vi "Mice staircase kinematics - MAIN.vi"() -> ()   [LabVIEW 2020]
panel:
  in  "FPS":dbl
  in  "Synergy data":string
  in  "Path length data":string
  in  "Velocity, acceleration graphs":string
  in  "Velocity, acceleration, smoothness data":string
  in  "Angle graphs":string
  in  "Angle data":string
  in  "Position graph":string
  in  "Position data":string
  out "Shoulder-Elbow angle data":dbl[][](array[numeric])
  out "Vel, Acc data":dbl[][](array[numeric])
  out "Angle-angle synergygrap":i32[][](array[numeric])
  out "Angle-angle synergy":dbl[][](array[numeric])
  out "Pos, Neg increments Position":dbl[][](array[numeric])
  out "Synergy Graph":i32[][](array[numeric])
  out "Synergy%":i32[][](array[numeric])
  out "Vel, Accel RMS":dbl[][](array[numeric])
  out "Path length data":dbl[][](array[numeric])
  in  "Step":dbl
  in  "Animal Number":dbl
  out "#Crossings":i32[][](array[numeric])
  out "Velocity-Acceleration graphs":dbl[][](array[numeric])
  out "Raw position":dbl[][](array[numeric])
  out "Pos, Neg increments":dbl[][](array[numeric])
  out "Elbow CircStat":dbl[](array[numeric])
  out "Shoulder CircStat Counterclockwise":dbl[](array[numeric])
  out "Angle RMS":dbl[][](array[numeric])
  out "Angle mean subtracted (output)":dbl[][](array[numeric])
  out "RMS":dbl[][](array[numeric])
  out "Normalized Position":dbl[][](array[numeric])
  out "Position (output)":dbl[][](array[numeric])
  # "The post-stroke hemiplegic rodent evaluation"
  # "FILE NAMES (DATA)"
  # "MAIN CONTROLS"
  # "DATA"
  # "FILE NAMES (GRAPHS)"
  # "GRAPHS"
  # "LabVIEW code by Gustavo Balbinot & Clarissa Pedrini Schuch"
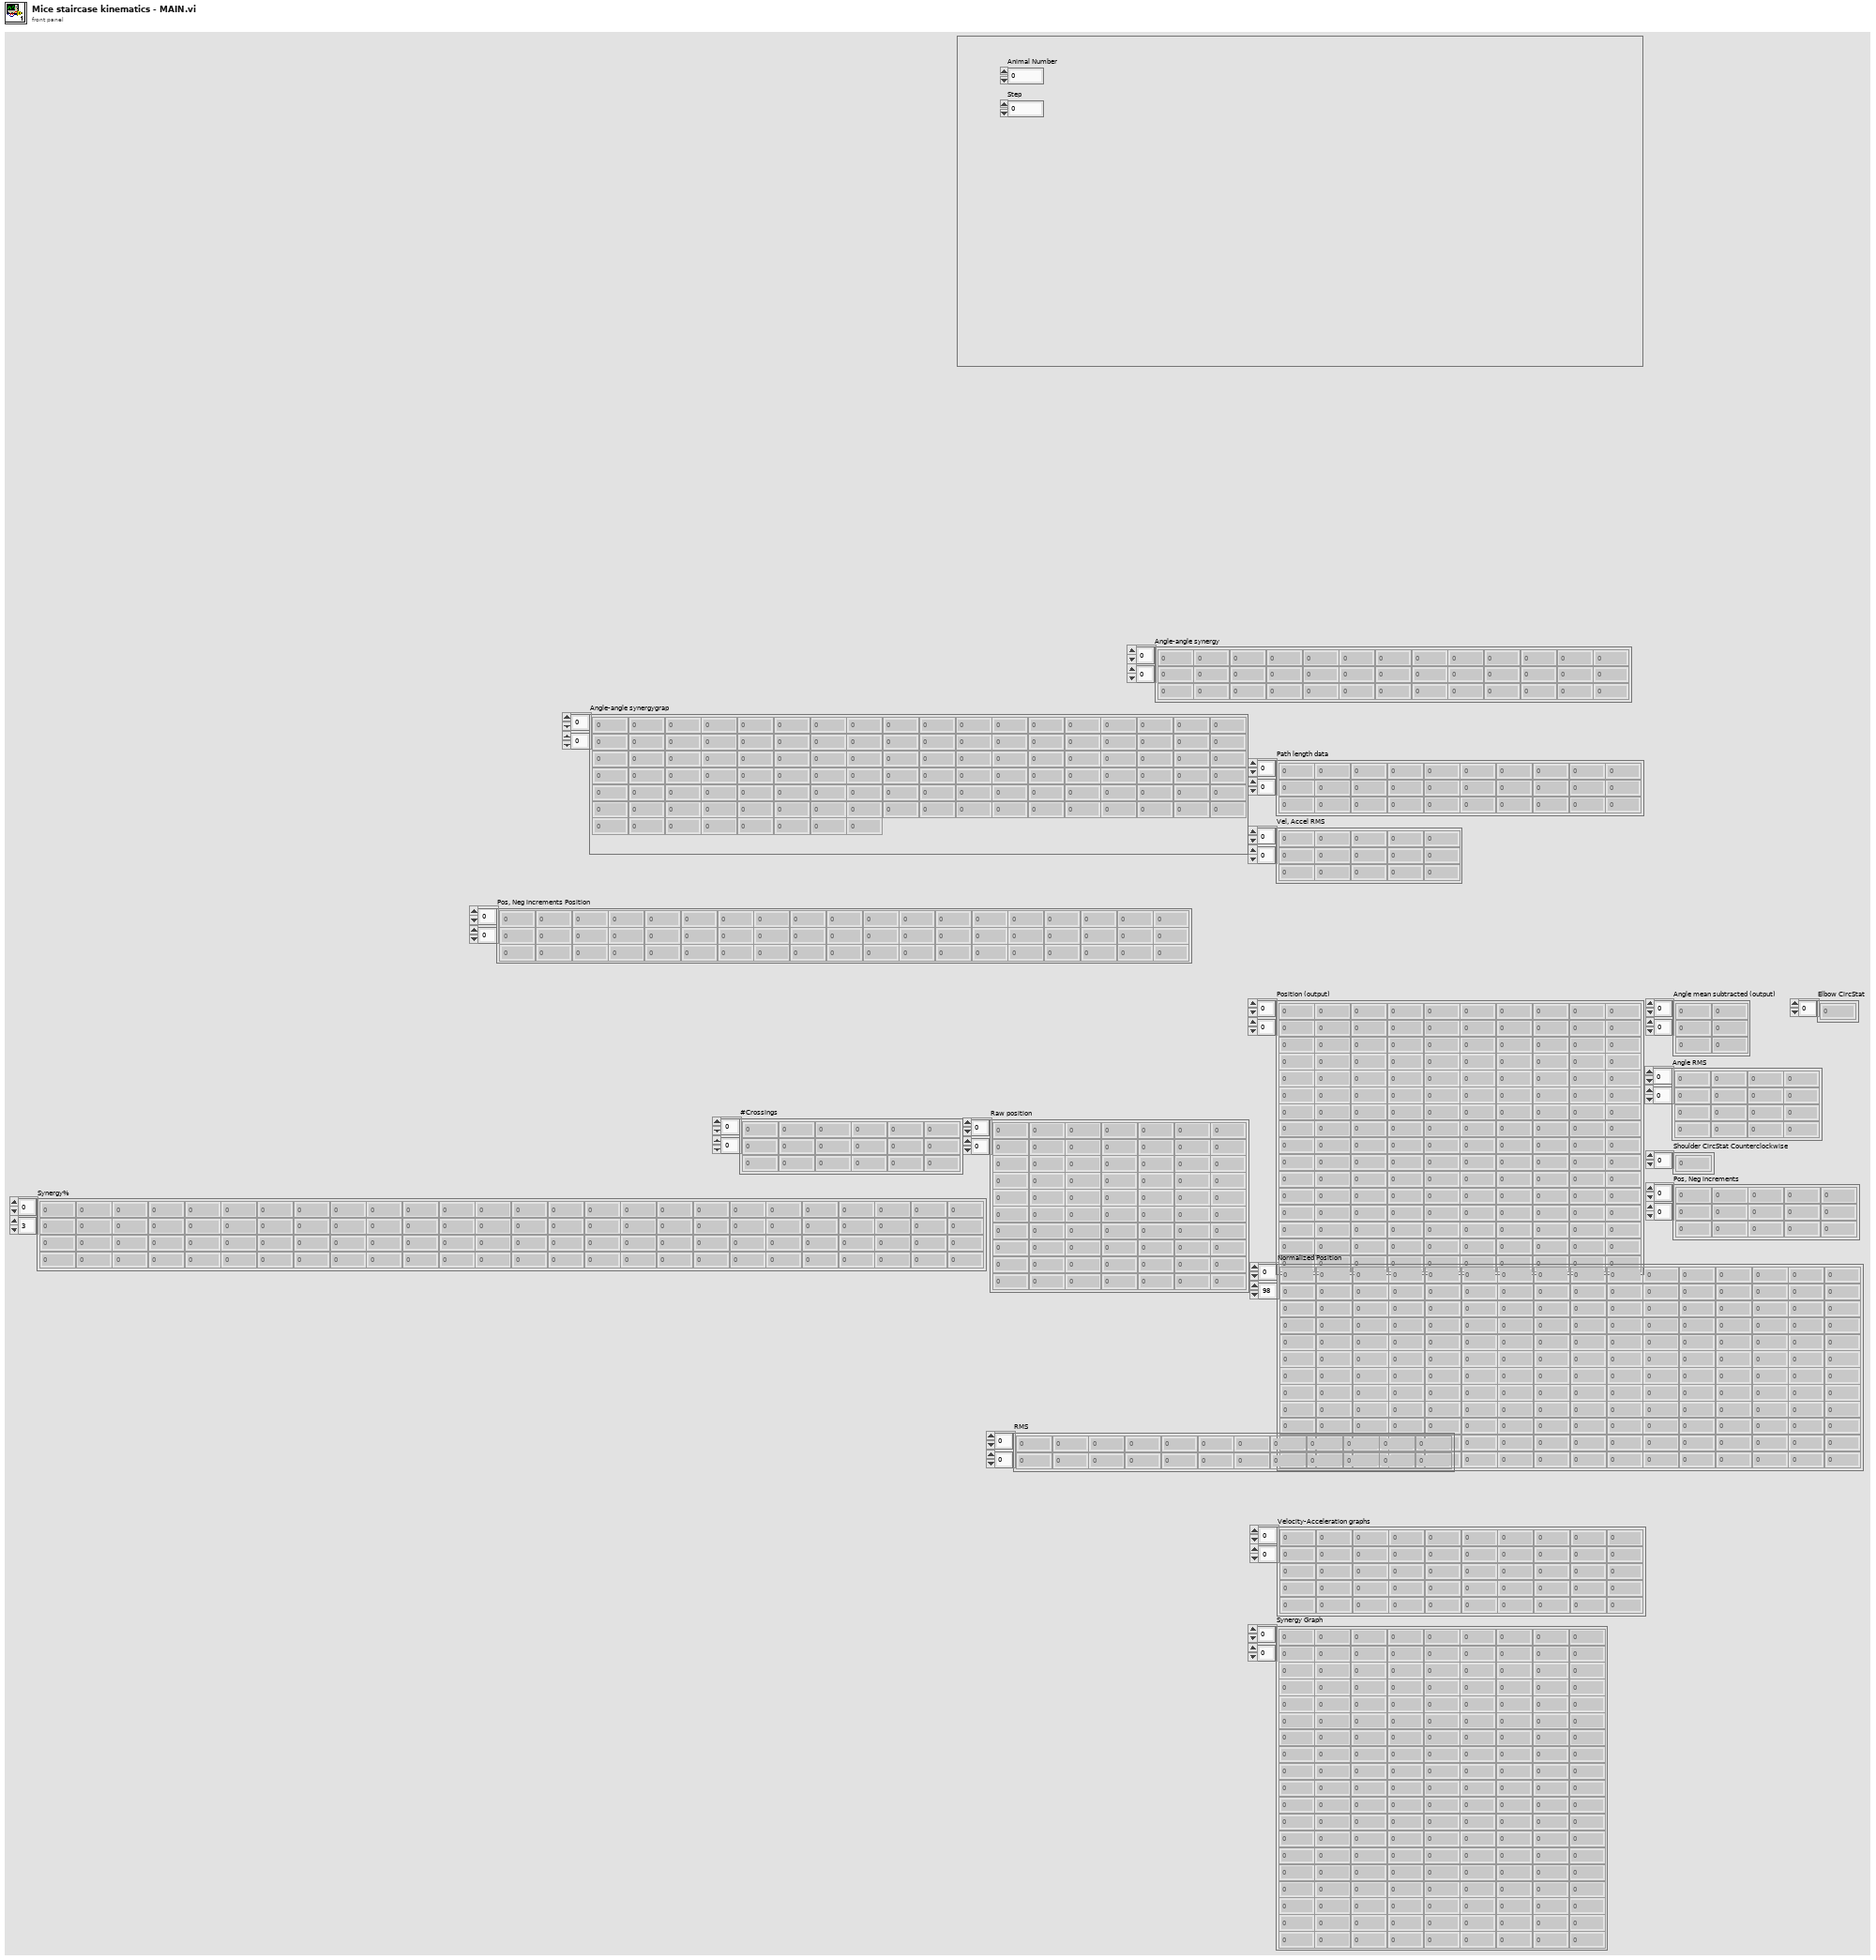
[diagram p1: front panel]
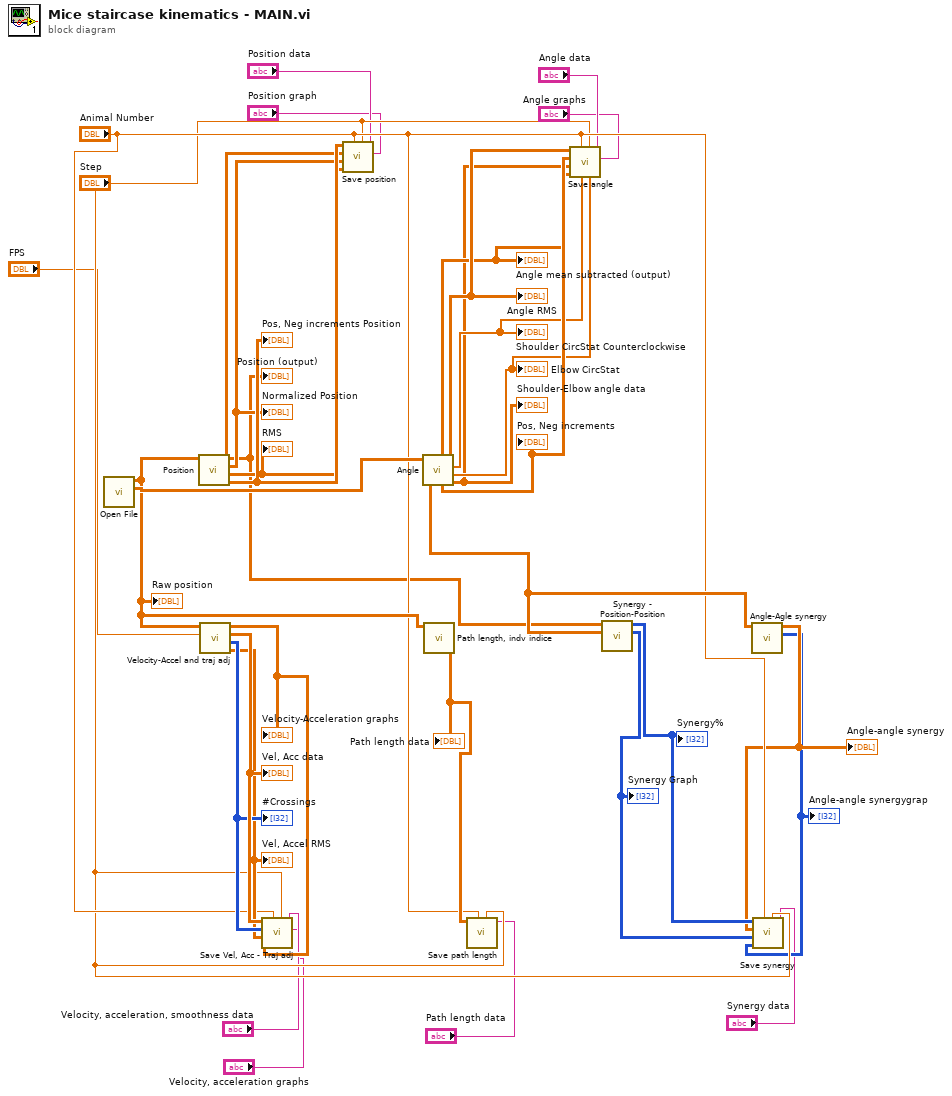
[diagram p0: block diagram]
diagram:
  n1 = call "Open File.vi"() -> ("Angle"=w33:dbl[][], "Position"=w32:dbl[][])  [unwired: 10 in]
  "Raw position" <- w32
  n2 = call "Position.vi"("Position"=w32) -> ("Position (output)"=w10:dbl[][], "Normalized Position"=w29:dbl[][], "RMS"=w28:dbl[][], "Pos, Neg increments Position"=w30:dbl[][])  [unwired: 5 in]
  "Position (output)" <- w10
  "Normalized Position" <- w29
  "RMS" <- w28
  "Pos, Neg increments Position" <- w30
  n3 = call "Velocity-Accel and traj adj.vi"("FPS"="FPS", "Raw position"=w32) -> ("Vel, Accel RMS"=w23:dbl[][], "#Crossings"=w24:i32[][], "Vel, Acc data"=w25:dbl[][], "Velocity-Acceleration graphs"=w18:dbl[][])  [unwired: 6 in]
  "Velocity-Acceleration graphs" <- w18
  "#Crossings" <- w24
  "Vel, Accel RMS" <- w23
  "Vel, Acc data" <- w25
  n4 = call "Save Vel, Acc - Traj adj.vi"("Vel,Acc graphs"="Velocity, acceleration graphs", "Vel,Acc traj Adj data"="Velocity, acceleration, smoothness data", "Step"="Step", "Animal Number"="Animal Number", "Velocity-Acceleration graphs"=w18, "Vel, Accel RMS"=w23, "#Crossings"=w24, "Vel, Acc data"=w25) -> ()  [unwired: 4 in]
  n5 = call "Save position.vi"("Position Graph"="Position graph", "Position data"="Position data", "Step"="Step", "Animal Number"="Animal Number", "RMS"=w28, "Normalized Position"=w29, "Position (output)"=w10, "Pos, Neg increments Position"=w30) -> ()  [unwired: 4 in]
  n6 = call "Angle.vi"("Angle"=w33) -> ("Shoulder-Elbow angle data"=w19:dbl[][], "Pos, Neg increments"=w26:dbl[][], "Elbow CircStat"=w21:dbl[], "Shoulder CircStat Counterclockwise"=w22:dbl[], "Angle mean subtracted (output)"=w20:dbl[][], "Angle RMS"=w27:dbl[][], "Angle for Synergy analysis"=w31:dbl[][])  [unwired: 1 in]
  "Angle mean subtracted (output)" <- w20
  "Angle RMS" <- w27
  "Shoulder CircStat Counterclockwise" <- w22
  "Elbow CircStat" <- w21
  "Pos, Neg increments" <- w26
  "Shoulder-Elbow angle data" <- w19
  n7 = call "Path length, indv indice.vi"("Raw position"=w32) -> ("Path length data"=w17:dbl[][])  [unwired: 10 in]
  "Path length data" <- w17
  n8 = call "Save path length.vi"("Path Length data"="Path length data", "Step"="Step", "Animal Number"="Animal Number", "Path length data"=w17) -> ()  [unwired: 8 in]
  n9 = call "Save angle.vi"("Angle graphs"="Angle graphs", "Angle data"="Angle data", "Elbow CircStat"=w21, "Step"="Step", "Shoulder CircStat Counterclockwise"=w22, "Animal Number"="Animal Number", "Angle mean subtracted (output)"=w20, "Shoulder-Elbow angle data"=w19, "Pos, Neg increments"=w26, "Angle RMS"=w27) -> ()  [unwired: 2 in]
  n10 = call "Synergy - Position-Position.vi"("Angle for Synergy analysis"=w31, "Position (output)"=w10) -> ("Synergy Graph"=w12:i32[][], "Synergy%"=w14:i32[][])  [unwired: 8 in]
  "Synergy%" <- w14
  "Synergy Graph" <- w12
  n11 = call "Angle-Agle synergy.vi"("Angle for Synergy analysis"=w31) -> ("Angle-angle synergygrap"=w11:i32[][], "Angle-angle synergy"=w13:dbl[][])  [unwired: 9 in]
  "Angle-angle synergy" <- w13
  "Angle-angle synergygrap" <- w11
  n12 = call "Save synergy.vi"("Synergy data"="Synergy data", "Step"="Step", "Animal Number"="Animal Number", "Angle-angle synergygrap"=w11, "Synergy Graph"=w12, "Angle-angle synergy"=w13, "Synergy%"=w14) -> ()  [unwired: 5 in]
